vi "Save for Previous Version.vi"(8 "error in (no error)":errorcluster, 10 "LabVIEW Version":string, 11 "VI File in":refnum<class "VI File.lvclass">) -> (0 "error out":errorcluster, 1 "Errors":string, 2 "Warnings":string, 3 "VI File out":refnum<class "VI File.lvclass">)   [LabVIEW 2020, in "Save for Previous Version.lvlib" / "VI File.lvclass"]
uses:
  VI File.lvclass
  \\Mac\Home/JKI/GitHub/vipm-io/a-version-explorer-for-labview/experiments/save-for-previous-version/source/File/File.lvclass/File.lvclass
  File/File.lvclass/File.lvclass/File.ctl
  VI File.lvclass/VI File.ctl
  File/File.lvclass/Read Path.vi
  Read VI Refnum.vi
  LabVIEW File/LabVIEW File.lvclass
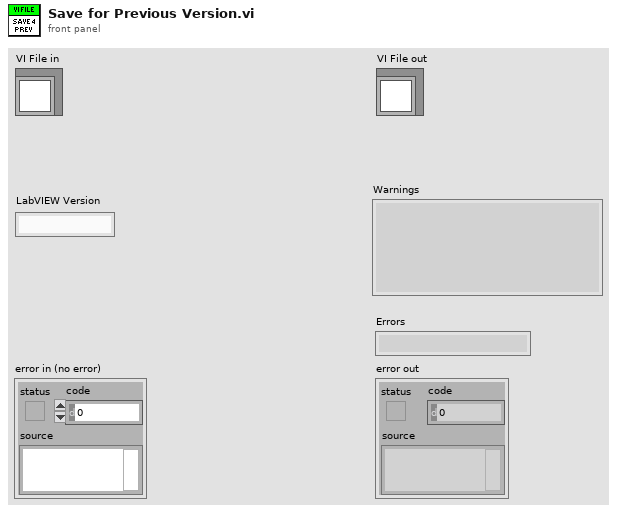
[diagram p1: front panel]
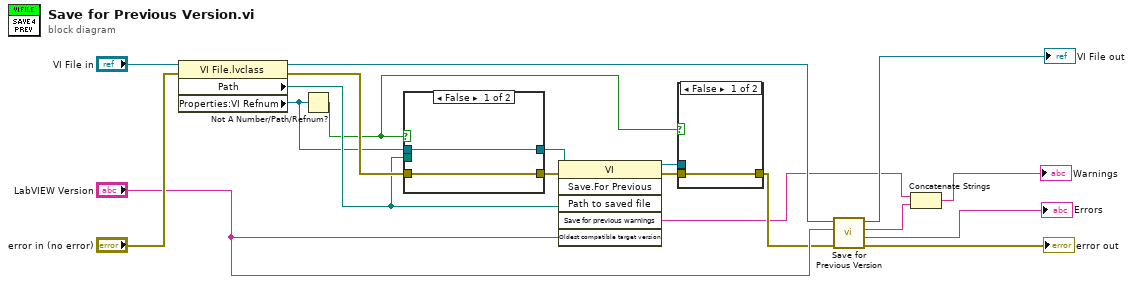
[diagram p0: block diagram]
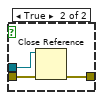
[diagram p2: hidden frame]
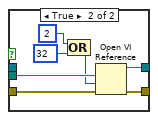
[diagram p3: hidden frame]
diagram:
  n1 = property class="VI File.lvclass"(reference="VI File in", error in="error in (no error)") -> (reference out=w19:refnum<class "VI File.lvclass">, error out=w10:errorcluster, "Path"=w3:path, "Properties:VI Refnum"=w2:refnum<vi>)
  n2 = Not A Number/Path/Refnum?(number/path/refnum=w2) -> (NaN/Path/Refnum?=w1:bool)
  n3 = case shown="False" w1 {
    tunnel: [w21 w28] -> w14
    tunnel: [w20 w27] -> w13
    tunnel: w10 -> [w20 w26]
    tunnel: w3 -> [_ w25]
    tunnel: w2 -> [w21 _]
    frame False {
    }
    frame True {
      n4 = Compound Arithmetic op=OR(2 ("options"), 32 ("options")) -> (w22:i32)
      n5 = Open VI Reference(vi path=w25, options=w22, error in (no error)=w26) -> (vi reference=w28:refnum<vi>, error out=w27:errorcluster)  [unwired: 3 in]
    }
  }
  n6 = invoke class="VI" method="Save.For Previous"(reference=w14, error in=w13, "Path to saved file"=w3, "Oldest compatible target version"="LabVIEW Version") -> (reference out=w11:refnum<vi>, error out=w12:errorcluster, "Save for previous warnings"=w6:string)  [unwired: 2 in, 3 out]
  n7 = case shown="False" w1 {
    tunnel: w12 -> [w29 w32]
    tunnel: w11 -> [_ w31]
    tunnel: [w29 w30] -> w8
    frame False {
    }
    frame True {
      n8 = Close Reference(reference=w31, error in (no error)=w32) -> (error out=w30:errorcluster)
    }
  }
  n9 = call-parent "Save for Previous Version.vi"("error in (no error)"=w8, "LabVIEW Version"="LabVIEW Version", "LabVIEW File in"=w19) -> ("error out"=→"error out":errorcluster, "Errors"=→"Errors":string, "Warnings"=w7:string, "LabVIEW File out"=→"VI File out":refnum<class "VI File.lvclass">)  [unwired: 5 in]
  n10 = Concatenate Strings(w6, w7) -> (→"Warnings":string)
